vi "Register Event Listener for Instances of A.vi"(7 "class A instances event ref":refnum<user-event>, 8 "error in (no error)":errorcluster, 11 "Lookup in":refnum<data-value>) -> (0 "error out":errorcluster, 3 "Lookup out":refnum<data-value>)   [LabVIEW 2014, in "LVCOOOP Tests.lvlib"]
uses:
  LVCOOOP Tests.lvlib
  LVCOOOP/Lookup API/Services/Lookup Service/Lookup Service.lvclass
  Base Class A.lvclass
  LVCOOOP/Lookup API/Providers/Default Lookup/Default Lookup.lvclass
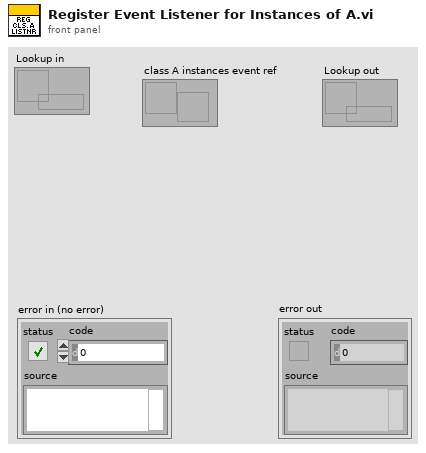
[diagram p1: front panel]
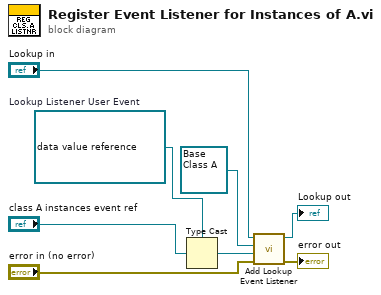
[diagram p0: block diagram]
diagram:
  w1 = refnum<user-event> refnum  # Lookup Listener User Event
  n1 = Type Cast(type=w1, x="class A instances event ref") -> (*(type *) &x=w6:refnum<user-event>)
  n2 = call "Add Lookup Event Listener.vi"("error in (no error)"="error in (no error)", "Lookup Listener User Event"=w6, "Base Class (LabVIEW Object)"=refnum<class "Base Class A.lvclass"> refnum ("LVCOOOP Tests.lvlib:Base Class A.lvclass"), "Lookup Service in"="Lookup in") -> ("error out"=→"error out":errorcluster, "Lookup Service out"=→"Lookup out":refnum<data-value>)  [unwired: 6 in]
